vi "Launcher.vi"   [LabVIEW 2012]
uses:
  <vilib>/ActorFramework/Actor/Actor.lvclass
  <vilib>/ActorFramework/Message Queue/Message Queue.lvclass
  DemoMain.lvclass
panel:
  # "Run me to launch"
  # "Run"
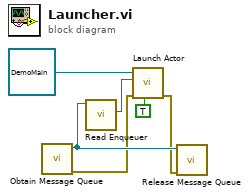
[diagram p0: block diagram]
diagram:
  n1 = call <vilib>:"Obtain Message Queue.vi"() -> ("error out"=w3:errorcluster, "Message Queue"=w4:refnum<class "Message Queue.lvclass">)  [unwired: 10 in]
  n2 = call <vilib>:"Read Enqueuer.vi"("Message Queue"=w4) -> ("Message Enqueuer"=w6:refnum<class "Message Enqueuer.lvclass">)  [unwired: 10 in]
  n3 = call <vilib>:"Launch Actor.vi"("Open Actor Core front panel? (F)"=TRUE, "error in (no error)"=w3, "Actor-to-Caller Enqueuer"=w6, "Actor"=refnum<class "DemoMain.lvclass"> refnum ("Win8uiDemo.lvlib:DemoMain.lvclass")) -> ("error out"=w2:errorcluster)  [unwired: 6 in, 1 out]
  n4 = call <vilib>:"Release Message Queue.vi"("error in (no error)"=w2, "Message Queue"=w4) -> ()  [unwired: 8 in, 2 out]
